vi "PantherLAB_Log - Convert DQMH Event.vi"(6 "New Event Type":T1, 9 "New Broadcast Name":string, 10 "Event Info (Converted)":T2={"Event VI Path"=path "", "Argument Path"=path "", "Wait Argument Path"=path "", "Event Arg Owner"=-1, "Event Name"="", "Type"=enum."Request"}, 11 "Module Info":T4) -> (0 "error out":errorcluster)   [LabVIEW 2016]
doc: "_____\nCreated using DQMH Framework: Event Scripter 7.1.0.1450."
uses:
  <vilib>/Delacor/Delacor QMH/Libraries/_Scripting Support/Module Info--cluster.ctl
  <vilib>/Delacor/Delacor QMH/Libraries/_Scripting Support/Module Type--enum.ctl
  <vilib>/Delacor/Delacor QMH/Libraries/_Scripting Support/Event Info (Existing)--cluster.ctl
  Program Files (x86)/National Instruments/LabVIEW 2016/project/Delacor/DQMH/_DQMH Remove Event/Event Type (All Permutations)--enum.ctl
  <vilib>/Delacor/Delacor QMH/Libraries/_Scripting Support/Event Type (Convert)--enum.ctl
  PantherLAB Scripting Hooks/PantherLAB_Scripting.lvlib
  <vilib>/Delacor/Delacor QMH/Libraries/_Scripting Support/dqmh_lib_DQMH Scripting Support.lvlib
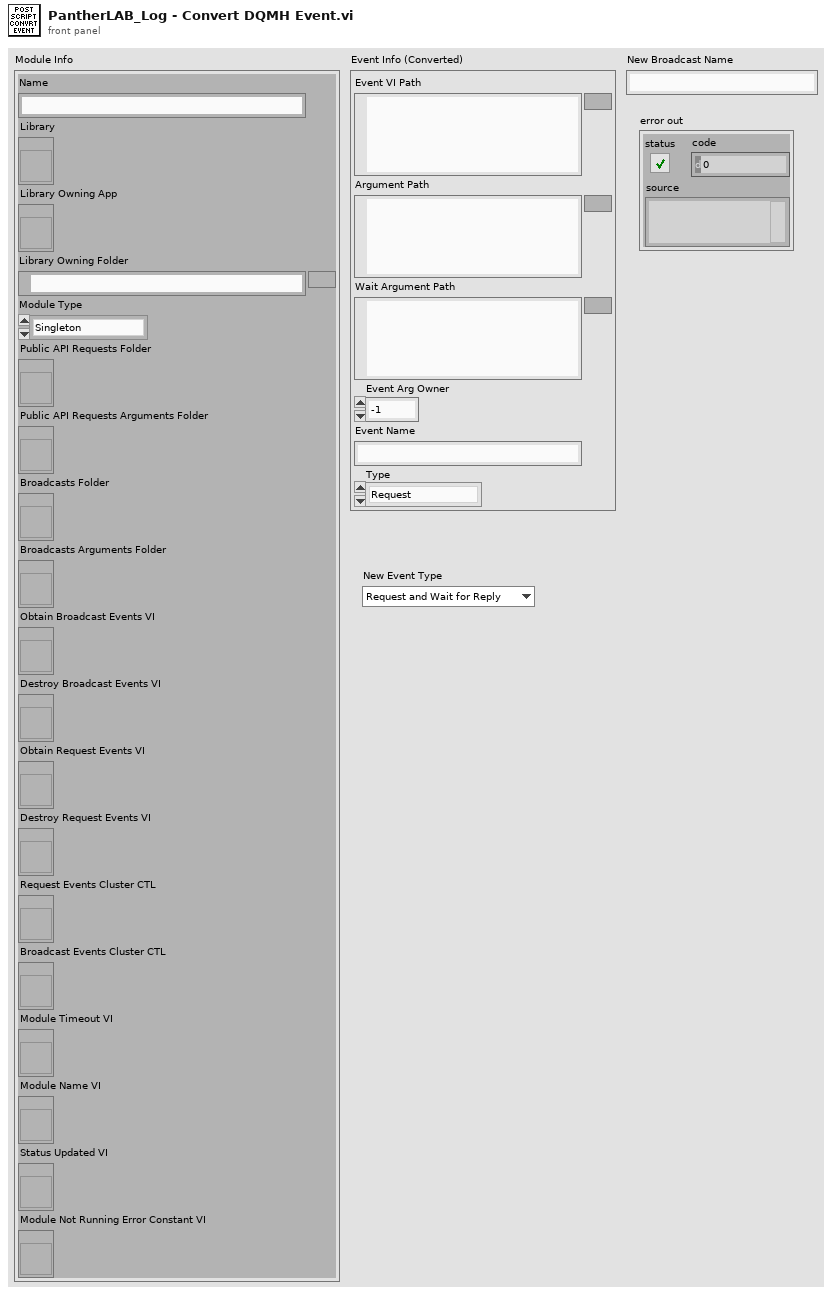
[diagram p1: front panel]
types:
  T1 = typedef "dqmh_lib_DQMH Scripting Support.lvlib/Event Type (Convert)--enum.ctl" = enum16{"Request and Wait for Reply", "Round Trip"}
  T2 = typedef "dqmh_lib_DQMH Scripting Support.lvlib/Event Info (Existing)--cluster.ctl" = cluster{"Event VI Path":path, "Argument Path":path, "Wait Argument Path":path, "Event Arg Owner":i32, "Event Name":string, "Type":T3}
  T3 = typedef "dqmh_lib_DQMH Scripting Support.lvlib/Event Type (All Permutations)--enum.ctl" = enum16{"Request", "Broadcast", "Both", "Request (no Wait)", "Request and Wait", "Request (Private)", "Request (Local Instance)"}
  T4 = typedef "dqmh_lib_DQMH Scripting Support.lvlib/Module Info--cluster.ctl" = cluster{"Name":string, "Library":refnum<vi>, "Library Owning App":refnum<vi>, "Library Owning Folder":path, "Module Type":T5, "Public API Requests Folder":refnum<vi>, "Public API Requests Arguments Folder":refnum<vi>, "Broadcasts Folder":refnum<vi>, "Broadcasts Arguments Folder":refnum<vi>, "Obtain Broadcast Events VI":refnum<vi>, "Destroy Broadcast Events VI":refnum<vi>, "Obtain Request Events VI":refnum<vi>, "Destroy Request Events VI":refnum<vi>, "Request Events Cluster CTL":refnum<vi>, "Broadcast Events Cluster CTL":refnum<vi>, "Module Timeout VI":refnum<vi>, "Module Name VI":refnum<vi>, "Status Updated VI":refnum<vi>, "Module Not Running Error Constant VI":refnum<vi>}
  T5 = typedef "dqmh_lib_DQMH Scripting Support.lvlib/Module Type--enum.ctl" = enum16{"Singleton", "Cloneable"}
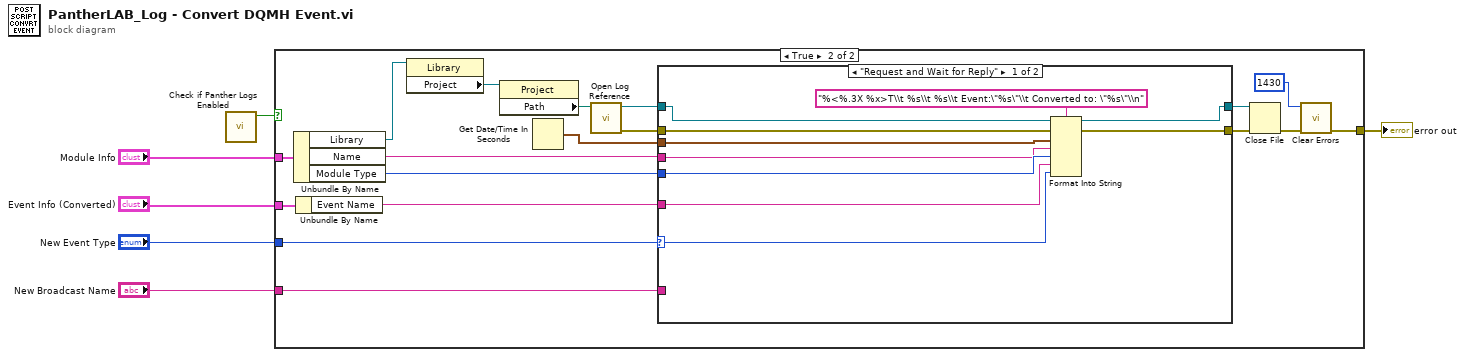
[diagram p0: block diagram]
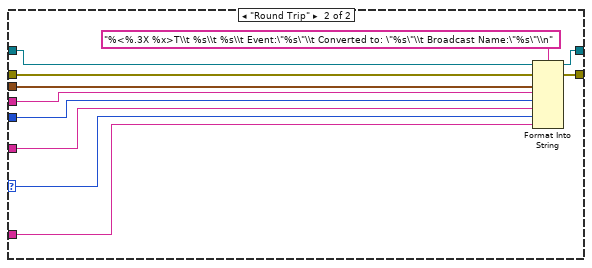
[diagram p3: hidden frame]
diagram:
  n1 = call "Check if Panther Logs Enabled.vi"() -> ("PantherLogs Enabled?"=w5:bool)  [unwired: 11 in]
  n2 = case shown="True" w5 {
    tunnel: [_ w8] -> w6
    tunnel: "Module Info" -> [_ w21]
    tunnel: "Event Info (Converted)" -> [_ w18]
    tunnel: "New Broadcast Name" -> [_ w10]
    tunnel: "New Event Type" -> [_ w11]
    frame False {
    }
    frame True {
      n3 = Unbundle By Name(w21) -> ("Library"=w20:refnum<vi>, "Name"=w15:string, "Module Type"=w14:T5)
      n4 = Unbundle By Name(w18) -> ("Event Name"=w9:string)
      n5 = property class="Library"(reference=w20) -> ("Project"=w19:refnum<vi>)  [unwired: 1 in, 2 out]
      n6 = property class="Project"(reference=w19) -> ("Path"=w12:path)  [unwired: 1 in, 2 out]
      n7 = Get Date/Time In Seconds() -> (seconds since 1Jan1904=w13:timestamp)
      n8 = call "Open Log Reference.vi"("Project Path"=w12) -> ("error out"=w24:errorcluster, "File Reference"=w17:refnum<file>)  [unwired: 9 in]
      n9 = case shown="\"Request and Wait for Reply\"" w11 {
        selector: w11 -> [w26 w37]
        tunnel: w17 -> [w32 w43]
        tunnel: w24 -> [w34 w45]
        tunnel: [w31 w42] -> w16
        tunnel: [w33 w44] -> w23
        tunnel: w15 -> [w29 w40]
        tunnel: w14 -> [w30 w41]
        tunnel: w13 -> [w28 w39]
        tunnel: w10 -> [_ w35]
        tunnel: w9 -> [w27 w38]
        frame "Request and Wait for Reply" {
          n10 = Format Into String(format string="%<%.3X %x>T\\t %s\\t %s\\t Event:\"%s\"\\t Converted to: \"%s\"\\n", initial string=w32, error in=w34, w28, w29, w30, w27, w26) -> (resulting string=w31:refnum<file>, error out=w33:errorcluster)
        }
        frame "Round Trip" {
          n11 = Format Into String(format string="%<%.3X %x>T\\t %s\\t %s\\t Event:\"%s\"\\t Converted to: \"%s\"\\t Broadcast Name:\"%s\"\\n", initial string=w43, error in=w45, w39, w40, w41, w38, w37, w35) -> (resulting string=w42:refnum<file>, error out=w44:errorcluster)
        }
      }
      n12 = Close File(refnum=w16, error in=w23) -> (error out=w22:errorcluster)  [unwired: 1 out]
      n13 = call <vilib>:"Clear Errors.vi"("error in (no error)"=w22, "specific error code to clear (0: all)"=1430) -> ("error out"=w8:errorcluster)  [unwired: 4 in, 1 out]
    }
  }
  "error out" <- w6
